vi "GarbageCollect.vi"   [LabVIEW 2020, in "ORM_API.lvlib"]
uses:
  ORM_API.lvlib
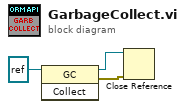
[diagram p0: block diagram]
diagram:
  n1 = invoke class="GC" method="Collect"(reference=refnum<k24> refnum) -> (reference out=w2:refnum<k24>, error out=w1:errorcluster)  [unwired: 2 in, 1 out]
  n2 = Close Reference(reference=w2, error in (no error)=w1) -> ()  [unwired: 1 out]
